vi "Initial Values-format and values-DBL.vi"() -> (1 "Values Array":dbl[](array[numeric]), 3 "Keys Array":T1)   [LabVIEW 2020]
uses:
  Typedefs/Ini file interface (DBL).ctl
  User Interface/Visualisation/Functional Imaging Viewer/Typedefs/Get-Set-Clear Control.ctl
  Global Variables/gl_UI Ctrl Refs.vi
  User Interface/Visualisation/Timelapse Viewer/Globals/gl_Time series viewer globals.vi
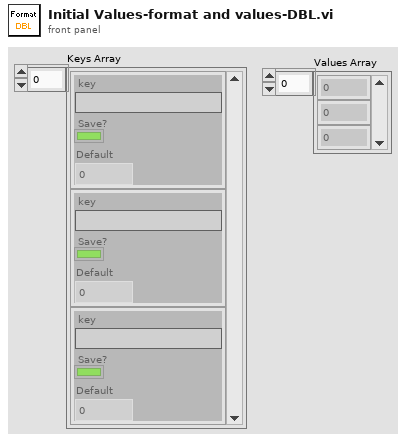
[diagram p1: front panel]
types:
  T1 = typedef "Ini file interface (DBL).ctl" = cluster{"key":string, "Save?":bool, "Default":dbl}[]
  T2 = typedef "Get-Set-Clear Control.ctl" = enum16{"Get", "Set", "Clear"}
  T3 = typedef "UI ctrl refs cluster.ctl" = cluster{"Top level VI path":path, "Top level VI ref":refnum<vi>, "User menu ref":refnum<k9>, "Sub Panel control":refnum<vi>, "Imaging Param Tab":refnum<vi>, "Occurrence-Start drivers":refnum<k4>, "Occurrence-Speed logging initialised":refnum<k4>, "Occurrence-XYZ stage initialised":refnum<k4>, "Exit button":refnum<vi>, "Status ind":refnum<vi>, "Set as origin":refnum<vi>, "Speed Logging":refnum<vi>, "Time Lapse":refnum<vi>, "Live Imaging":refnum<vi>, "AOL Z Stack":refnum<vi>, "Motor Z Stack":refnum<vi>, "Funct Acq button":refnum<vi>, "Hard Shutter":refnum<vi>, "Virtual Shutter":refnum<vi>, "Laser Power":refnum<vi>, "AOL Mode":refnum<vi>, "Frame Size":refnum<vi>, "Field of View":refnum<vi>, "Dwell Time":refnum<vi>, "Zoom":refnum<vi>, "AOL Z":refnum<vi>, "Objective":refnum<vi>, "Axis":refnum<vi>, "Paths & Names":refnum<vi>, "Experiment folder path (ind.)":refnum<vi>, "Last State (Ind.)":refnum<vi>, "Averages":refnum<vi>, "Angle (degrees)":refnum<vi>, "X centre":refnum<vi>, "Y centre":refnum<vi>, "Plane Mode":refnum<vi>, "# Planes":refnum<vi>, "Z Start":refnum<vi>, "Z Stop":refnum<vi>, "Z Step":refnum<vi>, "PMT 1":refnum<vi>, "PMT 2":refnum<vi>, "Stage XYZ Position":refnum<vi>, "Pockels@Z Start":refnum<vi>, "Pockels@Z Stop":refnum<vi>, "Obtain Z Start":refnum<vi>, "Obtain Z Stop":refnum<vi>, "Live stim.trig.period":refnum<vi>, "Live stim.trig.enable":refnum<vi>, "Movement Correction":refnum<vi>, "Load Reference Image":refnum<vi>, "XY Stage Move":refnum<vi>, "MovCor Cluster":refnum<vi>, "RefDAQParam":refnum<vi>, "Funct. Acq. Pockels Modulation":refnum<vi>, "Ref Laser Power":refnum<vi>, "Enable Video Recording":refnum<vi>, "Video Record-Live Imaging":refnum<vi>, "Video Record-Funct acq":refnum<vi>, "Reference Source":refnum<vi>, "AOL Z-stack Chirps Ready (ind)":refnum<vi>, "Target time between mov.cor. ref triggers (ms)":refnum<vi>, "Funct. Acq. Ref frame save":refnum<vi>, "Tracking button":refnum<vi>, "Show ref plots window":refnum<vi>, "Center freq ind (nm)":refnum<vi>, "Pickup mode (ind)":refnum<vi>, "Logging queue (ind)":refnum<vi>, "Back aperture power (ind.)":refnum<vi>, "Power after objective (ind.)":refnum<vi>, "Switch user":refnum<vi>, "Ls1 Conn. Status":refnum<vi>, "Ls1Tuning Status":refnum<vi>, "Ls1 Faults":refnum<vi>, "Ls1 Connection":refnum<vi>, "Ls1 Mode":refnum<vi>, "Ls1 POWER [mW]":refnum<vi>, "Ls1Shutter":refnum<vi>, "Ls1 Wavelength":refnum<vi>, "Ls1 Note":refnum<vi>, "Ls1 Confirm Wav":refnum<vi>, "Ls1 PreChrp Prism1":refnum<vi>, "Ls1 PreChrp Prism2":refnum<vi>, "Ls1 wav top Ind":refnum<vi>, "Ls1 power top Ind":refnum<vi>, "Ls1 Pump peak Hold":refnum<vi>, "Ls1 Status Ind":refnum<vi>, "Ls1 wav cancel":refnum<vi>, "Experiment Type":refnum<vi>, "Biology Information":refnum<vi>, "Camera recording status":refnum<vi>}
  T4 = typedef "AOL_Globals.ctl" = cluster{"Imaging Protocol":T5, "Number of POI":u16, "Number of Miniscans":u16, "Number of Trials":u16, "Number of Cycles ":u64, "# Averaged Frames":u16, "Laser power (%)":u8, "Pockels (V)":dbl, "Acquisition Length (sec)":dbl, "Fill time (us)":dbl, "POI Dwell time (us)":dbl, "Miniscan Dwell time per pixel (us)":dbl, "PMT 1":dbl, "PMT 2":dbl, "Back Apperture (mA)":dbl, "Frame Size":T6, "Center Frequency":dbl, "Field of View (norm)":dbl, "DwellTime (us)":dbl, "Wavelength (nm)":dbl, "Zoom":dbl, "AOL Z":dbl, "AOL Mode":T7, "GridXY":dbl, "GridZ":dbl, "TriggerPeriod (sec)":dbl, "Number of Pixels in Miniscan":u16, "Experiment folder path":path, "X centre":dbl, "Y centre":dbl, "Angle (degrees)":dbl, "Plane Mode":T8, "Threshold":u16[], "Regenerate Chirps":bool, "Rectangle ROI length (pixels)":u16, "Rectangle ROI height (pixels)":u16, "AOD fill":u16, "StartupDelay":i32, "Samples Wait after Trigger":u16, "Slip Cycle":u32, "Add Cycle":bool, "Functional Mode":T9, "Z Start":dbl, "Z Stop":dbl, "# Planes":i32, "Total Pixels":i32, "Variable Miniscan Pixels":u16[], "Use Variable Length":bool, "Use Variable Resolution":bool, "Laser power (%) at Z Start":u8, "Laser power (%) at Z Stop":u8, "Ref Z Step":i8, "Ref Dwell Time (us)":dbl, "Field of View (um)":dbl}
  T5 = typedef "Imaging Protocols enum.ctl" = enum16{"AOL Z-Stack", "Motor Z Stack", "Functional Acquisition", "Single Plane Acquisition", "Volume Acquisition", "Live Imaging", "Live Plane Imaging", "Live Volume Imaging"}
  T6 = typedef "Frame Size.ctl" = u16
  T7 = typedef "AOL modes.ctl" = enum16{"Raster", "Structural", "Pointing", "Mini Scan", "Alignment"}
  T8 = typedef "Plane Mode.ctl" = u16
  T9 = typedef "Functional Mode.ctl" = enum16{"Point", "Line", "Patch", "Plane", "Volume"}
  T10 = typedef "Stitch layout spec cluster.ctl" = cluster{"Timelapse image":cluster{"Image position":T11}, "Cam 1":cluster{"Image position":T11}, "Cam 2":cluster{"Image position":T11}, "Cam 3":cluster{"Image position":T11}, "Cam 4":cluster{"Image position":T11}}
  T11 = typedef "Image stitching positions.ctl" = enum16{"Top left", "Top right", "Bottom left", "Bottom right", "Not used"}
  T12 = typedef "PMT control knob.ctl" = u16
  T13 = typedef "Custom slider-horisontal.ctl" = cluster{dbl, dbl}
  T14 = typedef "Speed graph behaviour enum.ctl" = enum16{"Scrolling data", "Scrolling cursor"}
  T15 = typedef "AVI implementation enum.ctl" = enum16{"AVI1", "AVI2"}
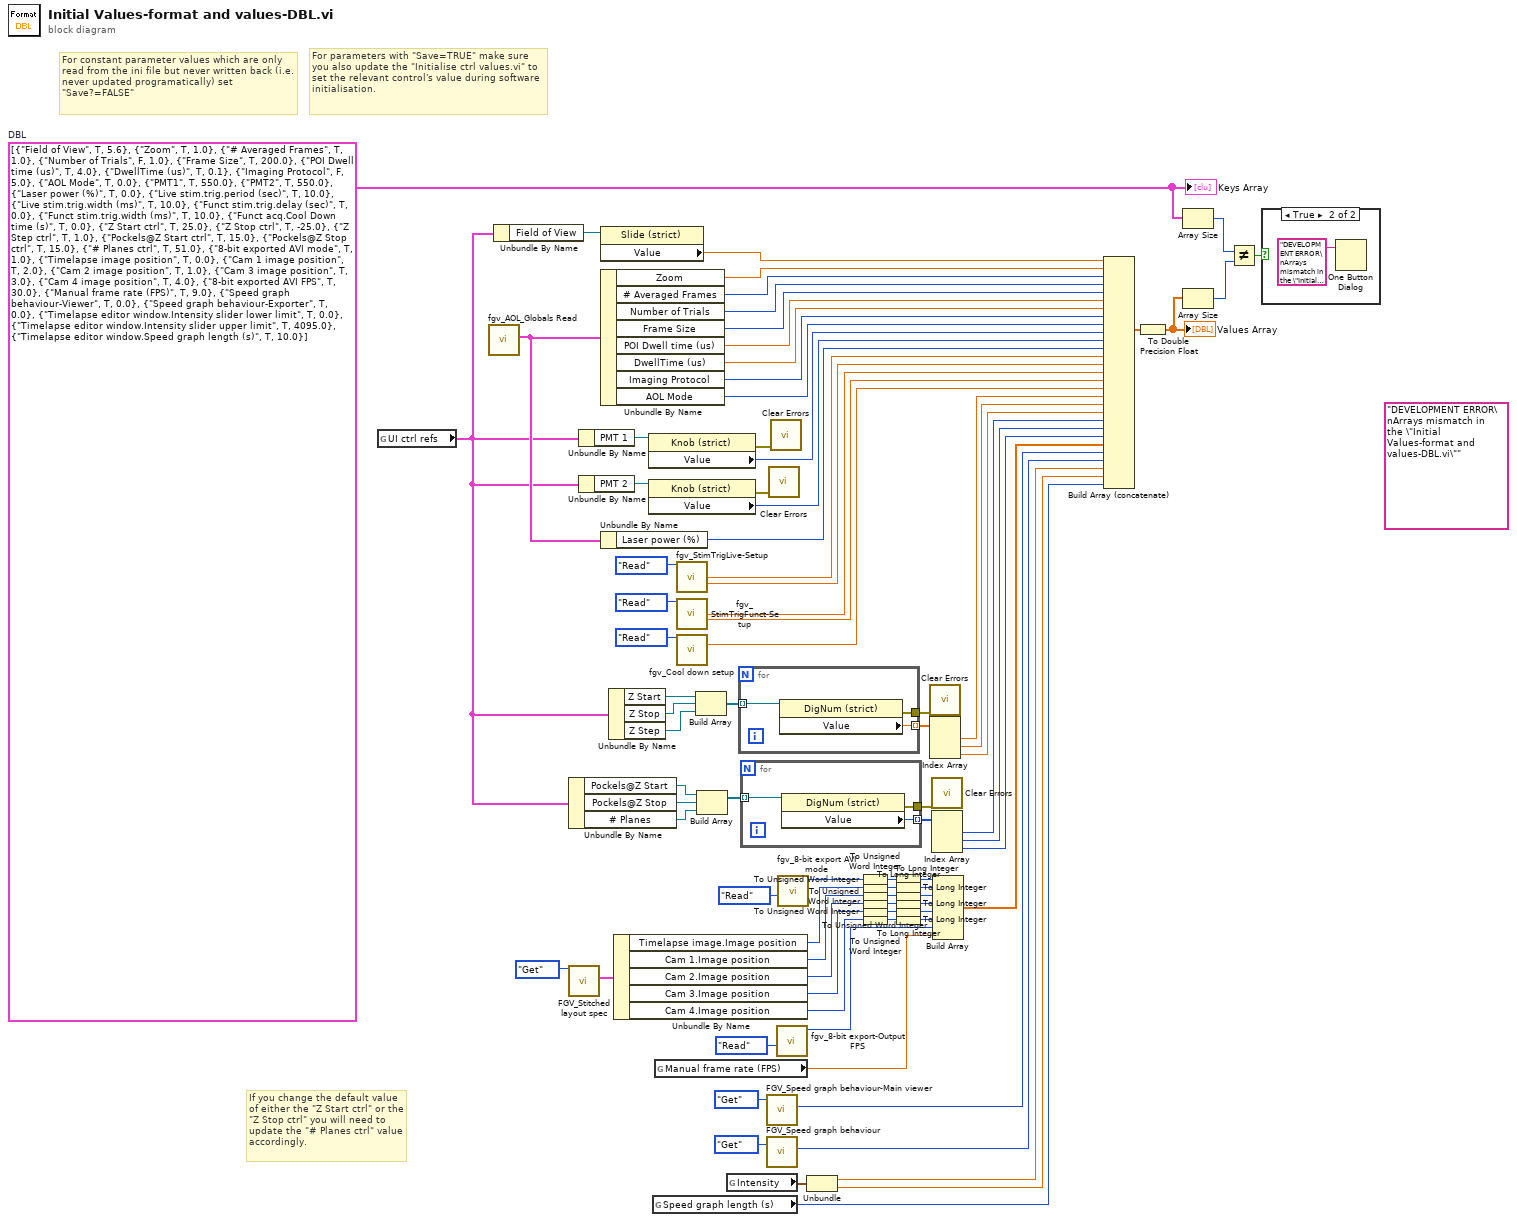
[diagram p0: block diagram]
diagram:
  (unwired) "DEVELOPMENT ERROR\nArrays mismatch in the \"Initial Values-format and values-DBL.vi\"" ("message")
  w58 = T1 [{"key"="Field of View", "Save?"=TRUE, "Default"=5.6}, {"key"="Zoom", "Save?"=TRUE, "Default"=1.0}, {"key"="# Averaged Frames", "Save?"=TRUE, "Default"=1.0}, {"key"="Number of Trials", "Save?"=FALSE, "Default"=1.0}, {"key"="Frame Size", "Save?"=TRUE, "Default"=200.0}, {"key"="POI Dwell time (us)", "Save?"=TRUE, "Default"=4.0}, {"key"="DwellTime (us)", "Save?"=TRUE, "Default"=0.1}, {"key"="Imaging Protocol", "Save?"=FALSE, "Default"=5.0}, {"key"="AOL Mode", "Save?"=TRUE, "Default"=0.0}, {"key"="PMT1", "Save?"=TRUE, "Default"=550.0}, {"key"="PMT2", "Save?"=TRUE, "Default"=550.0}, {"key"="Laser power (%)", "Save?"=TRUE, "Default"=0.0}, {"key"="Live stim.trig.period (sec)", "Save?"=TRUE, "Default"=10.0}, {"key"="Live stim.trig.width (ms)", "Save?"=TRUE, "Default"=10.0}, {"key"="Funct stim.trig.delay (sec)", "Save?"=TRUE, "Default"=0.0}, {"key"="Funct stim.trig.width (ms)", "Save?"=TRUE, "Default"=10.0}, {"key"="Funct acq.Cool Down time (s)", "Save?"=TRUE, "Default"=0.0}, {"key"="Z Start ctrl", "Save?"=TRUE, "Default"=25.0}, {"key"="Z Stop ctrl", "Save?"=TRUE, "Default"=-25.0}, {"key"="Z Step ctrl", "Save?"=TRUE, "Default"=1.0}, {"key"="Pockels@Z Start ctrl", "Save?"=TRUE, "Default"=15.0}, {"key"="Pockels@Z Stop ctrl", "Save?"=TRUE, "Default"=15.0}, {"key"="# Planes ctrl", "Save?"=TRUE, "Default"=51.0}, {"key"="8-bit exported AVI mode", "Save?"=TRUE, "Default"=1.0}, {"key"="Timelapse image position", "Save?"=TRUE, "Default"=0.0}, {"key"="Cam 1 image position", "Save?"=TRUE, "Default"=2.0}, {"key"="Cam 2 image position", "Save?"=TRUE, "Default"=1.0}, {"key"="Cam 3 image position", "Save?"=TRUE, "Default"=3.0}, {"key"="Cam 4 image position", "Save?"=TRUE, "Default"=4.0}, {"key"="8-bit exported AVI FPS", "Save?"=TRUE, "Default"=30.0}, {"key"="Manual frame rate (FPS)", "Save?"=TRUE, "Default"=9.0}, {"key"="Speed graph behaviour-Viewer", "Save?"=TRUE, "Default"=0.0}, {"key"="Speed graph behaviour-Exporter", "Save?"=TRUE, "Default"=0.0}, {"key"="Timelapse editor window.Intensity slider lower limit", "Save?"=TRUE, "Default"=0.0}, {"key"="Timelapse editor window.Intensity slider upper limit", "Save?"=TRUE, "Default"=4095.0}, {"key"="Timelapse editor window.Speed graph length (s)", "Save?"=TRUE, "Default"=10.0}]  # DBL
  # "If you change the default value of either the \"Z Start ctrl\" or the \"Z Stop ctrl\" you will need to update the \"# Planes ctrl\" value accordingly."
  # "For parameters with \"Save=TRUE\" make sure you also update the \"Initialise ctrl values.vi\" to set the relevant control's value during software initialisation."
  # "For constant parameter values which are only read from the ini file but never written back (i.e. never updated programatically) set \"Save?=FALSE\""
  n1 = global read "gl_UI Ctrl Refs.vi" "UI ctrl refs"() -> (w3:T3)
  n2 = call "fgv_AOL_Globals Read.vi"() -> ("AOL_Globals"=w71:T4)  [unwired: 9 in, 2 out]
  n3 = Unbundle By Name(w3) -> ("Field of View"=w2:refnum<vi>)
  n4 = Unbundle By Name(w3) -> ("Pockels@Z Start"=w48:refnum<vi>, "Pockels@Z Stop"=w49:refnum<vi>, "# Planes"=w40:refnum<vi>)
  n5 = call "FGV_Stitched layout spec.vi"("Function"=Get-Set-Clear_Control."Get") -> ("Stitch layout spec"=w34:T10)  [unwired: 9 in, 1 out]
  n6 = Unbundle By Name(w3) -> ("PMT 1"=w74:refnum<vi>)
  n7 = Unbundle By Name(w3) -> ("PMT 2"=w73:refnum<vi>)
  n8 = property class="Slide (strict)"(reference=w2) -> ("Value"=w1:sgl)  [unwired: 1 in, 2 out]
  n9 = Unbundle By Name(w71) -> ("Zoom"=w61:dbl, "# Averaged Frames"=w63:u16, "Number of Trials"=w62:u16, "Frame Size"=w64:T6, "POI Dwell time (us)"=w65:dbl, "DwellTime (us)"=w66:dbl, "Imaging Protocol"=w67:T5, "AOL Mode"=w68:T7)
  n10 = Unbundle By Name(w71) -> ("Laser power (%)"=w72:u8)
  n11 = Unbundle By Name(w3) -> ("Z Start"=w54:refnum<vi>, "Z Stop"=w52:refnum<vi>, "Z Step"=w51:refnum<vi>)
  n12 = Unbundle By Name(w34) -> ("Timelapse image.Image position"=w33:T11, "Cam 1.Image position"=w32:T11, "Cam 2.Image position"=w31:T11, "Cam 3.Image position"=w30:T11, "Cam 4.Image position"=w29:T11)
  n13 = property class="Knob (strict)"(reference=w74) -> (error out=w75:errorcluster, "Value"=w69:T12)  [unwired: 1 in, 1 out]
  n14 = property class="Knob (strict)"(reference=w73) -> (error out=w76:errorcluster, "Value"=w70:T12)  [unwired: 1 in, 1 out]
  n15 = global read "gl_Time series viewer globals.vi" "Speed graph length (s)"() -> (w4:i32)
  n16 = global read "gl_Time series viewer globals.vi" "Manual frame rate (FPS)"() -> (w15:dbl)
  n17 = call "fgv_StimTrigLive-Setup.vi"("Function"=enum16{"Intialize", "Write", "Read", "Clear"}."Read") -> ("Live stim.trig.period (sec)"=w79:dbl, "Live stim.trig.width (ms)"=w80:dbl)  [unwired: 11 in, 2 out]
  n18 = call "fgv_StimTrigFunct-Setup.vi"("Function"=enum16{"Intialize", "Write", "Read", "Clear"}."Read") -> ("Funct stim.trig.delay (sec)"=w81:dbl, "Funct stim.trig.width (ms)"=w82:dbl)  [unwired: 11 in, 2 out]
  n19 = call "fgv_Cool down setup.vi"("Function"=enum16{"Intialize", "Write", "Read", "Clear"}."Read") -> ("Cool-down time (s)"=w84:dbl)  [unwired: 12 in, 2 out]
  n20 = Build Array(w54, w52, w51) -> (w53:refnum<vi>[])
  n21 = Build Array(w48, w49, w40) -> (w46:refnum<vi>[])
  n22 = global read "gl_Time series viewer globals.vi" "Intensity"() -> (w7:T13)
  n23 = for {
    tunnel: w53 -> [w87] mode=indexing
    tunnel: [w86] -> w50 mode=indexing
    tunnel: [w85] -> w13
    n24 = property class="DigNum (strict)"(reference=w87) -> (error out=w85:errorcluster, "Value"=w86:dbl)  [unwired: 1 in, 1 out]
  }
  n25 = for {
    tunnel: w46 -> [w90] mode=indexing
    tunnel: [w89] -> w47 mode=indexing
    tunnel: [w88] -> w12
    n26 = property class="DigNum (strict)"(reference=w90) -> (error out=w88:errorcluster, "Value"=w89:u16)  [unwired: 1 in, 1 out]
  }
  n27 = call "FGV_Speed graph behaviour-Main viewer.vi"("Function"=Get-Set-Clear_Control."Get") -> ("Speed graph behaviour"=w9:T14)  [unwired: 9 in, 1 out]
  n28 = call "FGV_Speed graph behaviour.vi"("Function"=Get-Set-Clear_Control."Get") -> ("Speed graph behaviour"=w8:T14)  [unwired: 9 in, 1 out]
  n29 = call <vilib>:"Clear Errors.vi"("error in (no error)"=w76) -> ()  [unwired: 5 in, 2 out]
  n30 = call <vilib>:"Clear Errors.vi"("error in (no error)"=w75) -> ()  [unwired: 5 in, 2 out]
  n31 = call "fgv_8-bit export-Output FPS.vi"("Function"=enum16{"Intialize", "Write", "Read", "Clear"}."Read") -> ("Frames Per Second"=w38:u32)  [unwired: 9 in, 1 out]
  n32 = call "fgv_8-bit export AVI mode.vi"("Function"=enum16{"Intialize", "Write", "Read", "Clear"}."Read") -> ("AVI mode"=w36:T15)  [unwired: 9 in, 1 out]
  n33 = Unbundle(w7) -> (w6:dbl, w5:dbl)
  n34 = To Unsigned Word Integer(number=w36) -> (unsigned 16bit integer=w22:u16)
  n35 = To Unsigned Word Integer(number=w33) -> (unsigned 16bit integer=w21:u16)
  n36 = To Unsigned Word Integer(number=w32) -> (unsigned 16bit integer=w20:u16)
  n37 = To Unsigned Word Integer(number=w31) -> (unsigned 16bit integer=w19:u16)
  n38 = To Unsigned Word Integer(number=w30) -> (unsigned 16bit integer=w18:u16)
  n39 = To Unsigned Word Integer(number=w29) -> (unsigned 16bit integer=w17:u16)
  n40 = To Long Integer(number=w22) -> (32bit integer=w27:i32)
  n41 = To Long Integer(number=w21) -> (32bit integer=w28:i32)
  n42 = To Long Integer(number=w20) -> (32bit integer=w26:i32)
  n43 = To Long Integer(number=w19) -> (32bit integer=w25:i32)
  n44 = To Long Integer(number=w18) -> (32bit integer=w24:i32)
  n45 = To Long Integer(number=w17) -> (32bit integer=w23:i32)
  n46 = call <vilib>:"Clear Errors.vi"("error in (no error)"=w13) -> ()  [unwired: 5 in, 2 out]
  n47 = Index Array(array=w50) -> (element #1=w45:dbl, element #2=w44:dbl, element #3=w43:dbl)  [unwired: 3 in]
  n48 = call <vilib>:"Clear Errors.vi"("error in (no error)"=w12) -> ()  [unwired: 5 in, 2 out]
  n49 = Index Array(array=w47) -> (element #1=w42:u16, element #2=w41:u16, element #3=w39:u16)  [unwired: 3 in]
  n50 = Build Array(w27, w28, w26, w25, w24, w23, w38, w15) -> (w14:dbl[])
  n51 = Build Array (concatenate)(w1, w61, w63, w62, w64, w65, w66, w67, w68, w69, w70, w72, w79, w80, w81, w82, w84, w45, w44, w43, w42, w41, w39, w14, w9, w8, w6, w5, w4) -> (w60:dbl[])
  n52 = To Double Precision Float(number=w60) -> (double precision float=w59:dbl[])
  "Values Array" <- w59
  n53 = Array Size(array=w58) -> (size(s)=w57:i32)
  n54 = Array Size(array=w59) -> (size(s)=w56:i32)
  n55 = Not Equal?(x=w57, y=w56) -> (x != y?=w55:bool)
  n56 = case shown="True" w55 {
    frame False {
    }
    frame True {
      n57 = One Button Dialog(message="DEVELOPMENT ERROR\nArrays mismatch in the \"Initial Values-format and values-DBL.vi\"") -> ()  [unwired: 1 in, 1 out]
    }
  }
  "Keys Array" <- w58
